vi "Get Available Font Encoding [ ].vi"(5 "Font path":path=path "C:/Windows/Fonts/ARIALUNI.TTF", 7 "Encoding":string="Identity-H", 11 "error in (no error)":errorcluster) -> (6 "CodePagesSupported [ ]":string[](array[string])=["1252 Latin 1", "1250 Latin 2: Eastern Europe", "1251 Cyrillic", "1253 Greek", "1254 Turkish", "1255 Hebrew", "1256 Arabic", "1257 Windows Baltic", "1258 Vietnamese", "874 Thai", "932 JIS/Japan", "936 Chinese: Simplified chars--PRC and Singapore", "949 Korean Wansung", "950 Chinese: Traditional chars--Taiwan and Hong Kong", "1361 Korean Johab", "Macintosh Character Set (US Roman)", "OEM Character Set", "869 IBM Greek", "866 MS-DOS Russian", "865 MS-DOS Nordic", "864 Arabic", "863 MS-DOS Canadian French", "862 Hebrew", "861 MS-DOS Icelandic", "860 MS-DOS Portuguese", "857 IBM Turkish", "855 IBM Cyrillic; primarily Russian", "852 Latin 2", "775 MS-DOS Baltic", "737 Greek; former 437 G", "708 Arabic; ASMO 708", "850 WE/Latin 1", "437 US"], 8 "Number CodePagesSupported":i32=33, 15 "error out":errorcluster)   [LabVIEW 2019, in "Exaprom PDF.lvlib"]
doc: "Version 1.1\nDeveloped by Jean-Marc Simard\nCopyright © 2012, Exaprom Inc.\nAll rights reserved.\nLicense: BSD\n\nWith iTextSharp 4.1.6 (http://itextsharp.sourceforge.net)\nunder Mozilla Public License Version 1.1\n(http://www.mozilla.org/MPL/MPL-1.1.html)"
uses:
  C:/work/niobrara_lv/labview pdf writer fixing/DLL/itextsharp.dll
  DLL/itextsharp.dll
  Exaprom PDF.lvlib
panel:
  # "You nedd to know, at least, one encoding!"
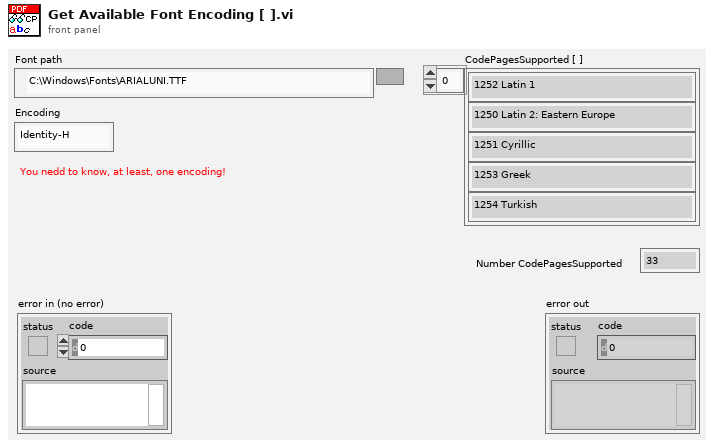
[diagram p1: front panel]
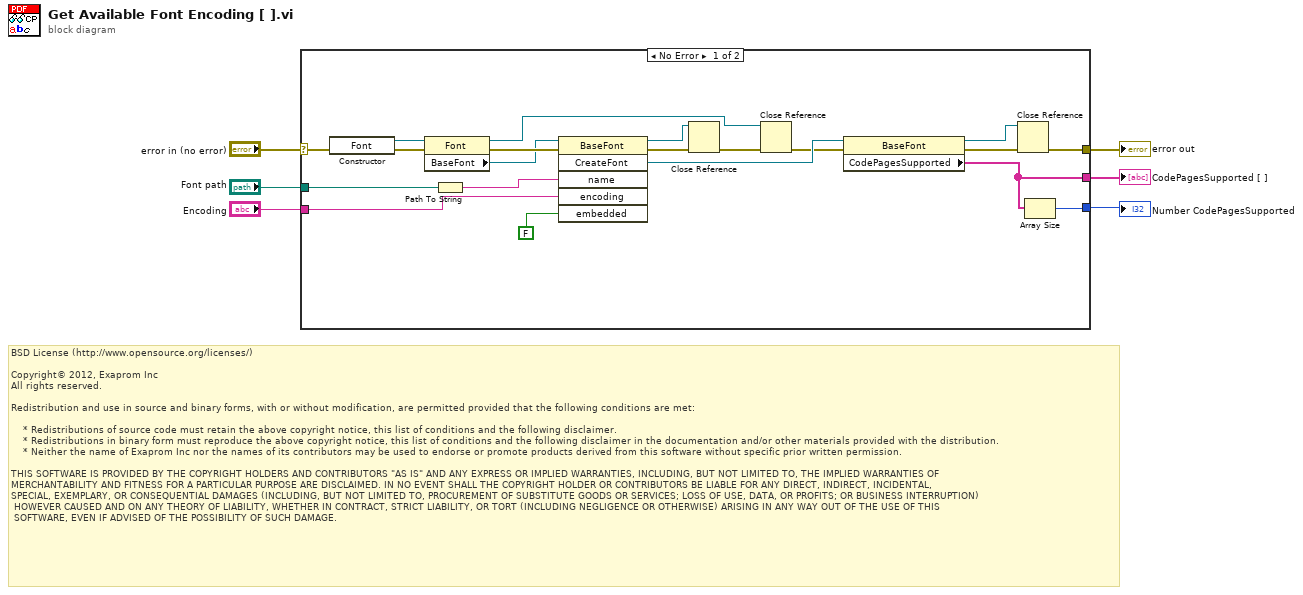
[diagram p0: block diagram]
diagram:
  # "BSD License (http://www.opensource.org/licenses/)\n\nCopyright© 2012, Exaprom Inc\nAll rights reserved.\n\nRedistribution and use in source and binary forms, with or without modification, are permitted provided that the following conditions are met:\n\n    * Redistributions of source code must retain the above copyright notice, this list of conditions and the following disclaimer.\n    * Redistributions in binary form must reproduce the above copyright notice, this list of conditions and the following disclaimer in the documentation and/or other materials provided with the distribution.\n    * Neither the name of Exaprom Inc nor the names of its contributors may be used to endorse or promote products derived from this software without specific prior written permission.\n\nTHIS SOFTWARE IS PROVIDED BY THE COPYRIGHT HOLDERS AND CONTRIBUTORS \"AS IS\" AND ANY EXPRESS OR IMPLIED WARRANTIES, INCLUDING, BUT NOT LIMITED TO, THE IMPLIED WARRANTIES OF \nMERCHANTABILITY AND FITNESS FOR A PARTICULAR PURPOSE ARE DISCLAIMED. IN NO EVENT SHALL THE COPYRIGHT HOLDER OR CONTRIBUTORS BE LIABLE FOR ANY DIRECT, INDIRECT, INCIDENTAL,\nSPECIAL, EXEMPLARY, OR CONSEQUENTIAL DAMAGES (INCLUDING, BUT NOT LIMITED TO, PROCUREMENT OF SUBSTITUTE GOODS OR SERVICES; LOSS OF USE, DATA, OR PROFITS; OR BUSINESS INTERRUPTION)\n HOWEVER CAUSED AND ON ANY THEORY OF LIABILITY, WHETHER IN CONTRACT, STRICT LIABILITY, OR TORT (INCLUDING NEGLIGENCE OR OTHERWISE) ARISING IN ANY WAY OUT OF THE USE OF THIS\n SOFTWARE, EVEN IF ADVISED OF THE POSSIBILITY OF SUCH DAMAGE."
  n1 = case shown="No Error" "error in (no error)" {
    selector: "error in (no error)" -> [w22 w27]
    tunnel: [w10 w27] -> w6
    tunnel: "Font path" -> [w20 _]
    tunnel: "Encoding" -> [w18 _]
    tunnel: [w12 _] -> w2
    tunnel: [w13 _] -> w1
    frame No Error {
      n2 = constructor class="Font"(error in=w22) -> (reference out=w26:refnum<k24>, error out=w25:errorcluster)  [unwired: 2 in, 1 out]
      n3 = property class="Font"(reference=w26, error in=w25) -> (reference out=w15:refnum<k24>, error out=w24:errorcluster, "BaseFont"=w8:refnum<k24>)
      n4 = Path To String(path=w20) -> (string=w19:string)
      n5 = invoke class="BaseFont" method="CreateFont"(reference=w8, error in=w24, "name"=w19, "encoding"=w18, "embedded"=FALSE) -> (reference out=w7:refnum<k24>, error out=w23:errorcluster, "CreateFont"=w21:refnum<k24>)  [unwired: 1 in, 3 out]
      n6 = Close Reference(reference=w7, error in (no error)=w23) -> (error out=w16:errorcluster)
      n7 = Close Reference(reference=w15, error in (no error)=w16) -> (error out=w14:errorcluster)
      n8 = property class="BaseFont"(reference=w21, error in=w14) -> (reference out=w9:refnum<k24>, error out=w11:errorcluster, "CodePagesSupported"=w12:string[])
      n9 = Close Reference(reference=w9, error in (no error)=w11) -> (error out=w10:errorcluster)
      n10 = Array Size(array=w12) -> (size(s)=w13:i32)
    }
    frame Error {
    }
  }
  "error out" <- w6
  "CodePagesSupported [ ]" <- w2
  "Number CodePagesSupported" <- w1
